vi "Set Edit Test Channel Sensor Names.vi"(8 "error in (no error)":errorcluster, 10 "Edit Test Channel Sensor Names":string[](array[string]), 11 "Abstract Edit Test Channel Sensor Names Msg in":refnum<class "Abstract Edit Test Channel Sensor Names Msg.lvclass">) -> (0 "error out":errorcluster, 3 "Abstract Edit Test Channel Sensor Names Msg out":refnum<class "Abstract Edit Test Channel Sensor Names Msg.lvclass">)   [LabVIEW 2013, in "Edit Test Channel Model.lvlib" / "Abstract Edit Test Channel Sensor Names Msg.lvclass"]
uses:
  Abstract Edit Test Channel Sensor Names Msg.lvclass
  Abstract Edit Test Channel Sensor Names Msg.lvclass/Abstract Edit Test Channel Sensor Names Msg.ctl
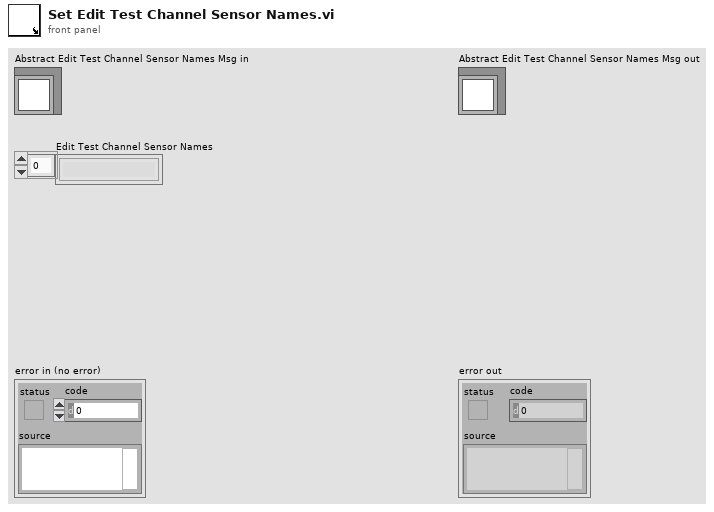
[diagram p1: front panel]
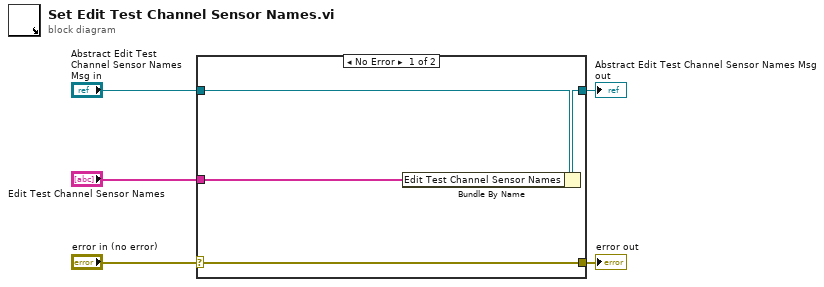
[diagram p0: block diagram]
diagram:
  n1 = case shown="No Error" "error in (no error)" {
    selector: "error in (no error)" -> [w9 w10]
    tunnel: [w9 w10] -> w4
    tunnel: [w7 w11] -> w2
    tunnel: "Abstract Edit Test Channel Sensor Names Msg in" -> [w8 w11]
    tunnel: "Edit Test Channel Sensor Names" -> [w6 _]
    frame No Error {
      n2 = Bundle By Name(cluster=w8, "Edit Test Channel Sensor Names"=w6) -> (w7:refnum<class "Abstract Edit Test Channel Sensor Names Msg.lvclass">)
    }
    frame Error {
    }
  }
  "error out" <- w4
  "Abstract Edit Test Channel Sensor Names Msg out" <- w2
